vi "FTW-ProjectItemManager-OwningProject.vi"(0 "Project Item Manager":refnum<class "FTW-ProjectItemManager.lvclass">, 11 "error in":errorcluster) -> (4 "Project Item Manager out":refnum<class "FTW-ProjectItemManager.lvclass">, 6 "Project":refnum<vi>, 15 "error out":errorcluster)   [LabVIEW 2012, in "FTW-ProjectItemManager.lvclass"]
uses:
  FTW-ProjectItemManager.lvclass
  FTW-ProjectItemManager.lvclass/FTW-ProjectItemManager.ctl
panel:
  # "Inputs"
  # "Outputs"
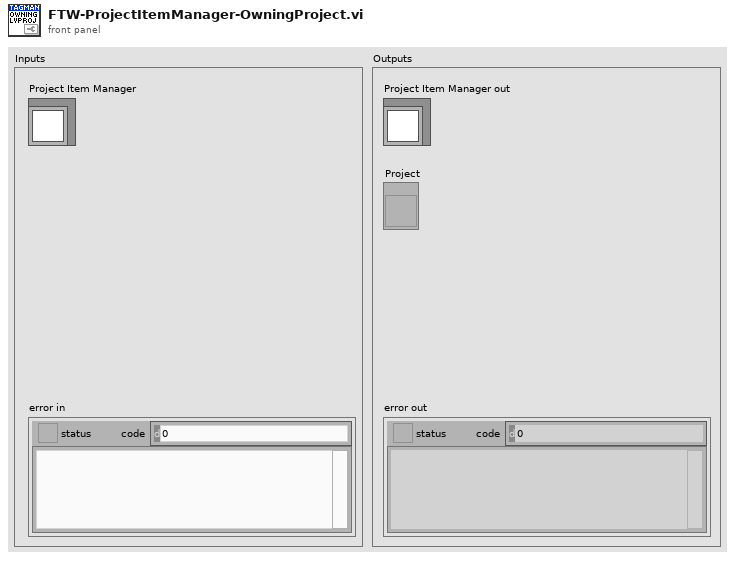
[diagram p1: front panel]
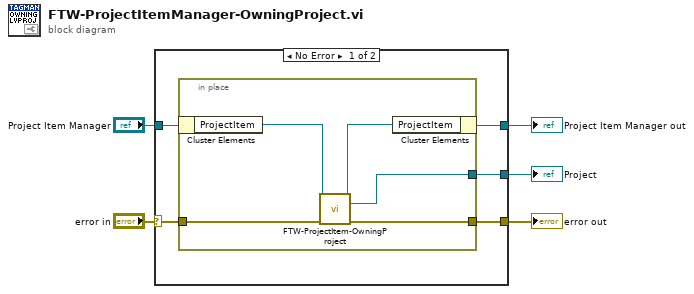
[diagram p0: block diagram]
diagram:
  n1 = case shown="No Error" "error in" {
    selector: "error in" -> [w9 w17]
    tunnel: [w7 w17] -> w5
    tunnel: [w8 w16] -> w3
    tunnel: "Project Item Manager" -> [w10 w16]
    tunnel: [w6 _] -> w1
    frame No Error {
      n2 = in-place {
        in-place-border: w9 -> [w13]
        in-place-border: [w12] -> w7
        in-place-border: [w11] -> w6
        n3 = in-place-cluster #1(w10) -> ("ProjectItem"=w15:refnum<vi>)
        n4 = call "FTW-ProjectItem-OwningProject.vi"("ProjectItem"=w15, "error in"=w13) -> ("ProjectItem out"=w14:refnum<vi>, "Project"=w11:refnum<vi>, "error out"=w12:errorcluster)  [unwired: 11 in]
        n5 = in-place-cluster #1("ProjectItem"=w14) -> (w8:refnum<class "FTW-ProjectItemManager.lvclass">)
      }
    }
    frame Error {
    }
  }
  "error out" <- w5
  "Project Item Manager out" <- w3
  "Project" <- w1
